vi "meta_writeFileBlock.vi"(8 "error in (no error)":errorcluster, 10 "meta_FileInfo":T4, 11 "meta file in":T1) -> (0 "error out":errorcluster, 3 "meta file out":T1)   [LabVIEW 2020, in "NI_ExcelFile.lvlib"]
uses:
  <vilib>/express/express shared/NI_ExcelFile/NI_ExcelFile.lvlib
  <vilib>/express/express shared/NI_ExcelFile/Ctrls/meta_FileInfo.ctl
  <vilib>/express/express shared/NI_ExcelFile/Ctrls/meta_FileInfo_2013.ctl
  <vilib>/express/express shared/NI_ExcelFile/Ctrls/FileAttribute.ctl
  <vilib>/express/express shared/NI_ExcelFile/Ctrls/meta_file.ctl
  <vilib>/express/express shared/NI_ExcelFile/Ctrls/meta_Block.ctl
  <vilib>/express/express shared/NI_ExcelFile/Ctrls/meta_BlockType.ctl
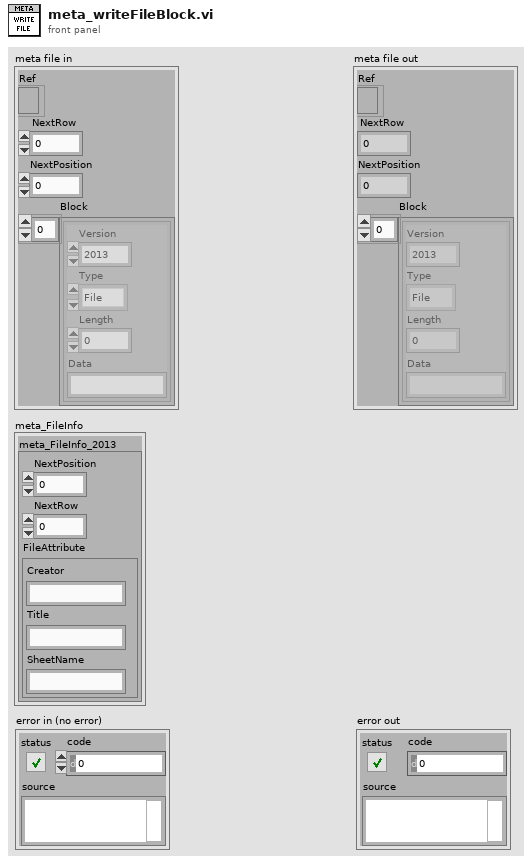
[diagram p1: front panel]
types:
  T1 = typedef "NI_ExcelFile.lvlib/meta_file.ctl" = cluster{"Ref":refnum<file>, "NextRow":i32, "NextPosition":i64, "Block":T2[]}
  T2 = typedef "NI_ExcelFile.lvlib/meta_Block.ctl" = cluster{"Version":u16, "Type":T3, "Length":i32, "Data":string}
  T3 = typedef "NI_ExcelFile.lvlib/meta_BlockType.ctl" = enum16{"NITag", "File", "Column"}
  T4 = typedef "NI_ExcelFile.lvlib/meta_FileInfo.ctl" = cluster{"meta_FileInfo_2013":T5}
  T5 = typedef "NI_ExcelFile.lvlib/meta_FileInfo_2013.ctl" = cluster{"NextPosition":i64, "NextRow":i32, "FileAttribute ":T6}
  T6 = typedef "NI_ExcelFile.lvlib/FileAttribute.ctl" = cluster{"Creator":string, "Title":string, "SheetName":string}
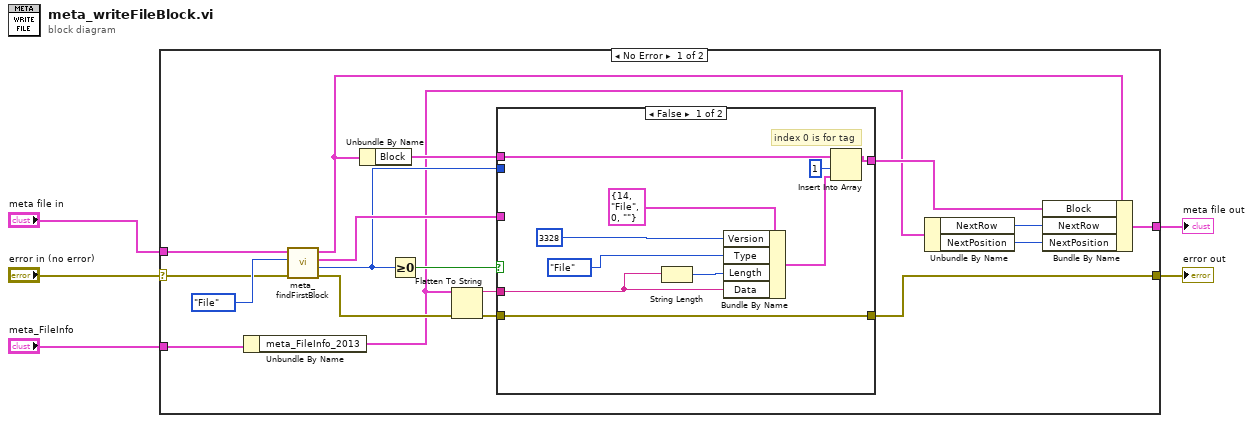
[diagram p0: block diagram]
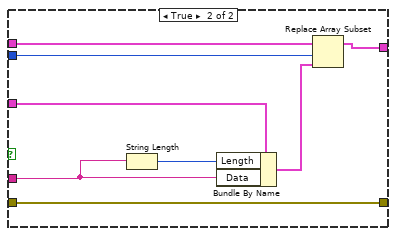
[diagram p2: hidden frame]
diagram:
  n1 = case shown="No Error" "error in (no error)" {
    selector: "error in (no error)" -> [w19 w43]
    tunnel: "meta_FileInfo" -> [w16 _]
    tunnel: [w22 w42] -> w4
    tunnel: "meta file in" -> [w18 w42]
    tunnel: [w15 w43] -> w2
    frame No Error {
      n2 = Unbundle By Name(w16) -> ("meta_FileInfo_2013"=w7:T5)
      n3 = call <vilib>:"meta_findFirstBlock.vi"("error in"=w19, "block type"=meta_BlockType."File", "meta file in"=w18) -> ("error out"=w8:errorcluster, "index"=w10:i32, "block out"=w11:T2, "meta file out"=w13:T1)  [unwired: 5 in]
      n4 = Unbundle By Name(w13) -> ("Block"=w14:T2[])
      n5 = Greater Or Equal To 0?(x=w10) -> (x >= 0?=w17:bool)
      n6 = Flatten To String(anything=w7, error in (no error)=w8) -> (data string=w6:string, error out=w9:errorcluster)  [unwired: 2 in, 1 out]
      n7 = case shown="False" w17 {
        tunnel: w9 -> [w26 w38]
        tunnel: [w26 w38] -> w15
        tunnel: w14 -> [w29 w41]
        tunnel: [w28 w39] -> w12
        tunnel: w11 -> [_ w37]
        tunnel: w10 -> [_ w40]
        tunnel: w6 -> [w27 w35]
        frame False {
          # "index 0 is for tag"
          n8 = String Length(string=w27) -> (length=w30:i32)
          n9 = Bundle By Name(cluster=T2 {"Version"=14, "Type"=enum."File", "Length"=0, "Data"=""} ("Block"), "Version"=u16 3328 ("version"), "Type"=meta_BlockType."File" ("type"), "Length"=w30, "Data"=w27) -> (w25:T2)
          n10 = Insert Into Array(array=w29, index=1, new element=w25) -> (w28:T2[])
        }
        frame True {
          n11 = String Length(string=w35) -> (length=w36:i32)
          n12 = Bundle By Name(cluster=w37, "Length"=w36, "Data"=w35) -> (w34:T2)
          n13 = Replace Array Subset(array=w41, new element=w34, index=w40) -> (w39:T2[])
        }
      }
      n14 = Unbundle By Name(w7) -> ("NextRow"=w21:i32, "NextPosition"=w20:i64)
      n15 = Bundle By Name(cluster=w13, "Block"=w12, "NextRow"=w21, "NextPosition"=w20) -> (w22:T1)
    }
    frame Error {
    }
  }
  "meta file out" <- w4
  "error out" <- w2
